vi "ListAvailableCOMPorts.vi"(8 "error in (no error)":errorcluster, 11 "VISA resource":string) -> (0 "error out":errorcluster, 2 "Available COM Ports":string[](array[string]))   [LabVIEW 2019]
uses:
  <vilib>/Instr/_visa.llb/VISA Find Search Mode.ctl
  GLOBALS.vi
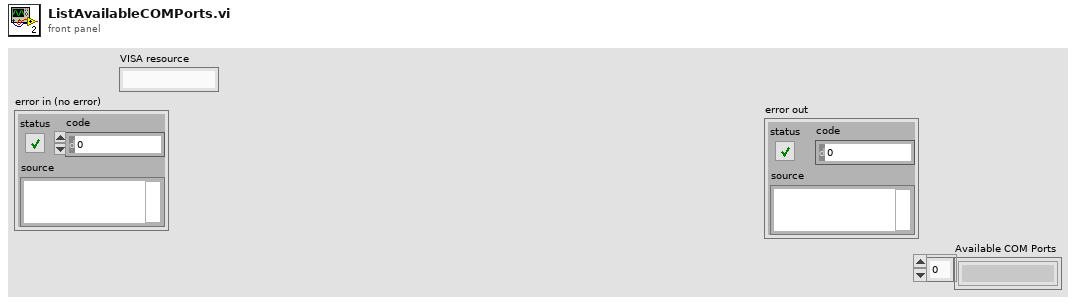
[diagram p1: front panel]
types:
  T1 = typedef "VISA Find Search Mode.ctl" = u32
  T2 = typedef "Globals_IO.ctl" = cluster{"Reserved COM ports":cluster{"Port":string, "Reserved By":string, "Time":timestamp}[]}
  T3 = cluster{"Port":string, "Reserved By":string, "Time":timestamp}[]
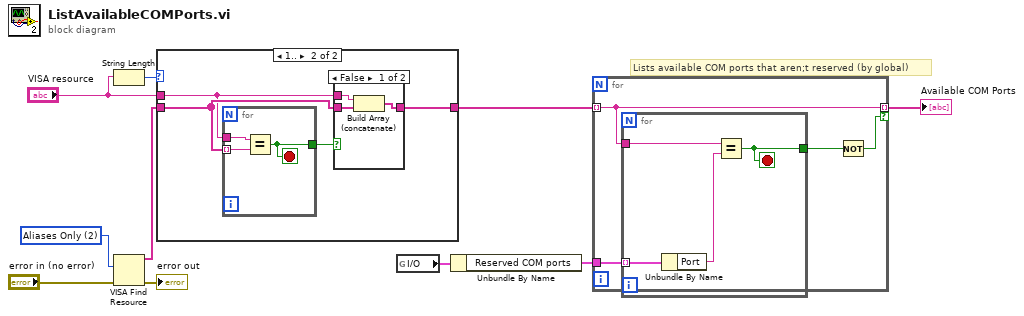
[diagram p0: block diagram]
diagram:
  w3 = T1 2 items=["Canonical Names Only"=0, "Aliases Only"=2, "Include Matching Aliases"=3, "Include All Aliases"=4] ("Search Mode")
  # "Lists available COM ports that aren;t reserved (by global)"
  n1 = String Length(string="VISA resource") -> (length=w7:i32)
  n2 = VISA Find Resource(8:"error in (no error)", 10:w3) -> (0:→"error out":errorcluster, 3:w9:string[])  [unwired: 1 in, 1 out]
  n3 = case shown="1.." w7 {
    tunnel: w9 -> [w11 w13]
    tunnel: [w11 w15] -> w8
    tunnel: "VISA resource" -> [_ w12]
    frame 0, Default {
    }
    frame 1.. {
      n4 = for {
        tunnel: w13 -> [w21] mode=indexing
        tunnel: w12 -> [w22]
        tunnel: [w20] -> w14
        stop <- w20 stop-if-true
        n5 = Equal?(x=w22, y=w21) -> (x = y?=w20:bool)
      }
      n6 = case shown="False" w14 {
        tunnel: [w18 w19] -> w15
        tunnel: w13 -> [w17 w19]
        tunnel: w12 -> [w16 _]
        frame False {
          n7 = Build Array (concatenate)(w16, w17) -> (w18:string[])
        }
        frame True {
        }
      }
    }
  }
  n8 = global read "Globals.vi" "I/O"() -> (w6:T2)
  n9 = Unbundle By Name(w6) -> ("Reserved COM ports"=w5:T3)
  n10 = for {
    tunnel: w8 -> [w25] mode=indexing
    tunnel: w5 -> [w26]
    tunnel: [w25] -> w4 mode=indexing if=w23
    n11 = for {
      tunnel: w25 -> [w30]
      tunnel: w26 -> [w28] mode=indexing
      tunnel: [w29] -> w24
      stop <- w29 stop-if-true
      n12 = Unbundle By Name(w28) -> ("Port"=w27:string)
      n13 = Equal?(x=w30, y=w27) -> (x = y?=w29:bool)
    }
    n14 = Not(x=w24) -> (.not. x?=w23:bool)
  }
  "Available COM Ports" <- w4
